vi "DSF.Memory.Buffer.Get Channel Props Pointer.vi"(8 "error in (no error)":errorcluster, 11 "Buffer in":refnum<class "DSF.Memory.Buffer.lvclass">) -> (0 "error out":errorcluster, 2 "Channel Properties pointer":refnum<class "DSF.Memory.Pointer.Channel Properties.lvclass">, 3 "Buffer out":refnum<class "DSF.Memory.Buffer.lvclass">)   [LabVIEW 2016, in "DSF.Memory.lvlib" / "DSF.Memory.Buffer.lvclass"]
uses:
  DSF.Memory.Buffer.lvclass
  Memory.Pointer/DSF.Memory.Pointer.Channel Properties.lvclass
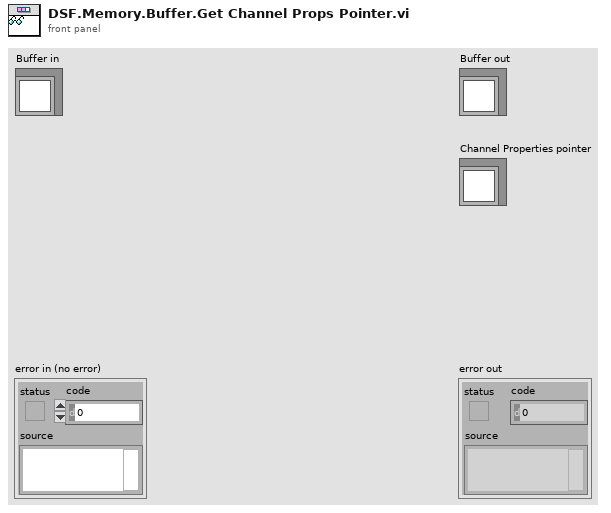
[diagram p1: front panel]
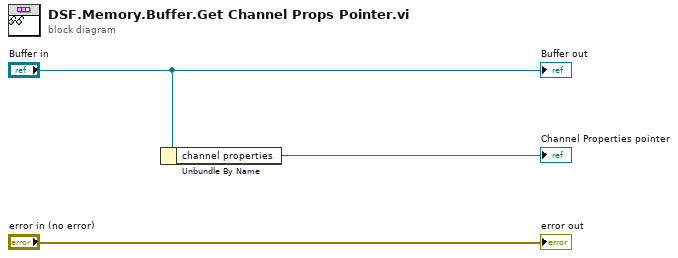
[diagram p0: block diagram]
diagram:
  n1 = Unbundle By Name("Buffer in") -> ("channel properties"=→"Channel Properties pointer":refnum<class "DSF.Memory.Pointer.Channel Properties.lvclass">)
  "error out" <- "error in (no error)"
  "Buffer out" <- "Buffer in"
